vi "Treshold.vi"() -> ()   [LabVIEW 2012]
uses:
  <vilib>/Instr/_visa.llb/VISA Configure Serial Port (Instr).vi
  Globalna_Variabla.vi
panel:
  out "Threshold float value":dbl
  in  "Baud Rate (9600)":u32=9600
  in  "VISA resource name":refnum<visa-resource-name>="COM18"
  in  "Reciving Byte Count (9)":u32=20
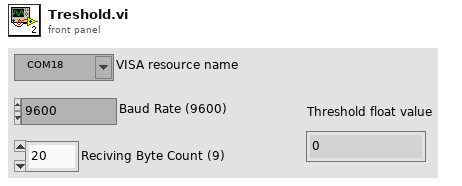
[diagram p1: front panel]
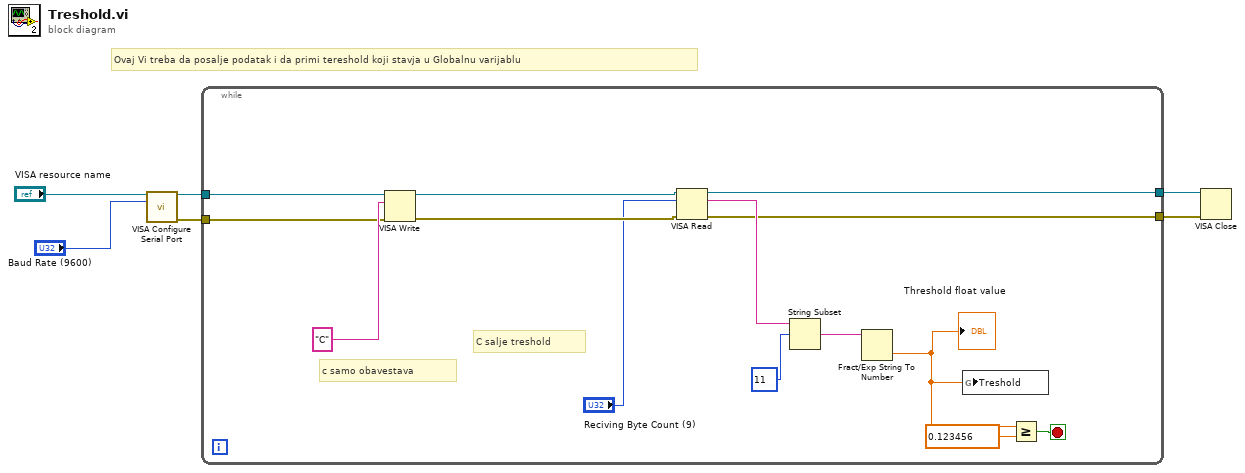
[diagram p0: block diagram]
diagram:
  # "Ovaj Vi treba da posalje podatak i da primi tereshold koji stavja u Globalnu varijablu"
  n1 = call-poly "VISA Configure Serial Port"("VISA resource name"="VISA resource name", "baud rate (9600)"="Baud Rate (9600)") -> ("VISA resource name out"=w4:refnum<visa-resource-name>, "error out"=w3:errorcluster)  [unwired: 12 in]
  n2 = while {
    tunnel: w4 -> [w18]
    tunnel: w3 -> [w17]
    tunnel: [w11] -> w2
    tunnel: [w10] -> w1
    stop <- w20 stop-if-true
    # "C salje treshold"
    # "c samo obavestava"
    n3 = VISA Write(VISA resource name=w18, write buffer="C", error in (no error)=w17) -> (VISA resource name out=w13:refnum<visa-resource-name>, error out=w12:errorcluster)  [unwired: 1 out]
    n4 = VISA Read(VISA resource name=w13, byte count="Reciving Byte Count (9)", error in (no error)=w12) -> (VISA resource name out=w11:refnum<visa-resource-name>, read buffer=w15:string, error out=w10:errorcluster)  [unwired: 1 out]
    n5 = String Subset(string=w15, offset (0)=11) -> (substring=w16:string)  [unwired: 1 in]
    n6 = Fract/Exp String To Number(string=w16) -> (number=w8:dbl)  [unwired: 3 in, 1 out]
    "Threshold float value" <- w8
    n7 = global write "Globalna_Variabla.vi" "Treshold"(w8) -> ()
    n8 = Greater Or Equal?(x=w8, y=0.123456) -> (x >= y?=w20:bool)
  }
  n9 = VISA Close(VISA resource name=w2, error in (no error)=w1) -> ()  [unwired: 1 out]
